vi "LookupECUPin.vi"(7 "Socket":u32, 10 "ECU Pin":string="DUT0_SignalName_Pin2", 11 "LookupTable":refnum<data-value>) -> (0 "error out":errorcluster, 2 "key not found?":bool, 3 "Info":T1)   [LabVIEW 2024, in "Shared Steps.lvlib"]
doc: "Lookup the test rack IO based on ECU pin and Socket."
uses:
  Shared Steps.lvlib
  Types/Pin Mapping.ctl
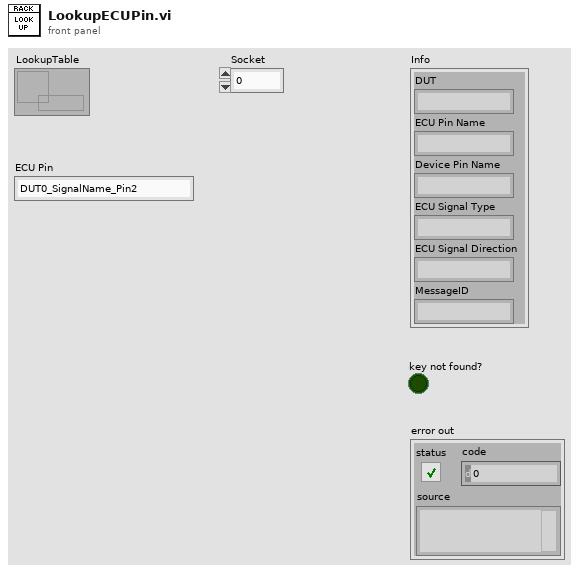
[diagram p1: front panel]
types:
  T1 = typedef "Shared Steps.lvlib/Pin Mapping.ctl" = cluster{"DUT":string, "ECU Pin Name":string, "Device Pin Name":string, "ECU Signal Type":string, "ECU Signal Direction":string, "MessageID":string}
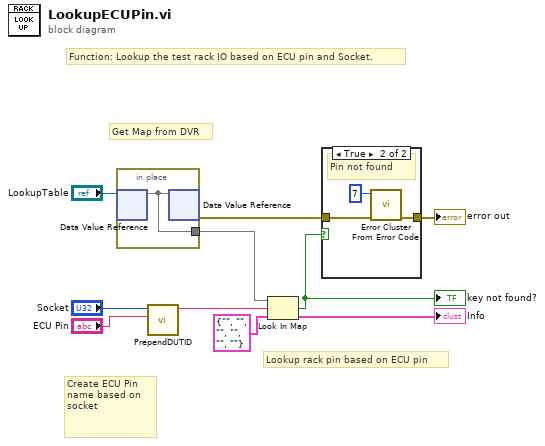
[diagram p0: block diagram]
diagram:
  # "Function: Lookup the test rack IO based on ECU pin and Socket."
  # "Lookup rack pin based on ECU pin"
  # "Create ECU Pin name based on socket"
  # "Get Map from DVR"
  n1 = in-place {
    in-place-border: [w11] -> w8
    n2 = in-place-dvr #1("LookupTable") -> (w11:map{string, T1})  [unwired: 1 out]
    n3 = in-place-dvr #1(w11) -> (w6:errorcluster)  [unwired: 1 out]
  }
  n4 = call "PrependDUTID.vi"("ECU Pin"="ECU Pin", "Socket"="Socket") -> ("String"=w1:string)  [unwired: 9 in]
  n5 = Look In Map(map=w8, key=w1, default value=T1 {"DUT"="", "ECU Pin Name"="", "Device Pin Name"="", "ECU Signal Type"="", "ECU Signal Direction"="", "MessageID"=""} ("cluster")) -> (key not found?=w7:bool, value=→"Info":T1)
  "key not found?" <- w7
  n6 = case shown="True" w7 {
    tunnel: [w12 w14] -> w9
    tunnel: w6 -> [w12 w13]
    frame False {
    }
    frame True {
      # "Pin not found"
      n7 = call <vilib>:"Error Cluster From Error Code.vi"("error in (no error)"=w13, "error code (0)"=7) -> ("error out"=w14:errorcluster)  [unwired: 7 in]
    }
  }
  "error out" <- w9
